vi "reorder roi.vi"(9 "Cluster Cursori":T1, 10 "Peak":i32, 11 "List ROI In in":dbl[][](array[numeric])) -> (2 "invert?":bool, 3 "List ROI In out":dbl[][](array[numeric]))   [LabVIEW 2023]
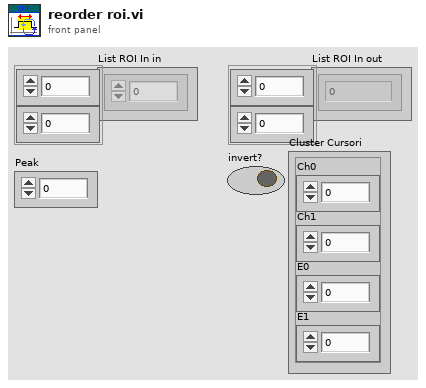
[diagram p1: front panel]
types:
  T1 = cluster{"Ch0":dbl, "Ch1":dbl, "E0":dbl, "E1":dbl}
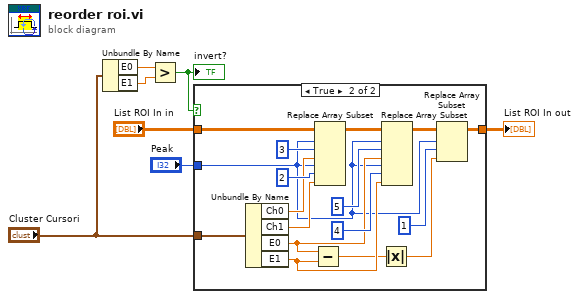
[diagram p0: block diagram]
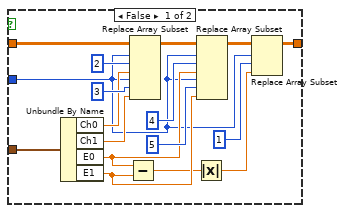
[diagram p2: hidden frame]
diagram:
  n1 = Unbundle By Name("Cluster Cursori") -> ("E0"=w2:dbl, "E1"=w1:dbl)
  n2 = Greater?(x=w2, y=w1) -> (0:w4:bool)
  "invert?" <- w4
  n3 = case shown="True" w4 {
    tunnel: "List ROI In in" -> [w24 w41]
    tunnel: [w8 w25] -> w6
    tunnel: "Peak" -> [w10 w27]
    tunnel: "Cluster Cursori" -> [w20 w37]
    frame False {
      n4 = Unbundle By Name(w20) -> ("Ch0"=w19:dbl, "Ch1"=w18:dbl, "E0"=w15:dbl, "E1"=w14:dbl)
      n5 = Subtract(x=w15, y=w14) -> (x-y=w13:dbl)
      n6 = Replace Array Subset(array=w24, new element #1=w19, index (row) #1=w10, index (col) #1=2, new element #2=w18, index (row) #2=w10, index (col) #2=3) -> (w23:dbl[][])
      n7 = Absolute Value(x=w13) -> (abs(x)=w11:dbl)
      n8 = Replace Array Subset(array=w23, new element #1=w15, index (row) #1=w10, index (col) #1=4, new element #2=w14, index (row) #2=w10, index (col) #2=5) -> (w12:dbl[][])
      n9 = Replace Array Subset(array=w12, new element=w11, index (row)=w10, index (col)=1 ("disabled index (col)")) -> (w8:dbl[][])
    }
    frame True {
      n10 = Unbundle By Name(w37) -> ("Ch0"=w36:dbl, "Ch1"=w35:dbl, "E0"=w32:dbl, "E1"=w31:dbl)
      n11 = Subtract(x=w32, y=w31) -> (x-y=w30:dbl)
      n12 = Replace Array Subset(array=w41, new element #1=w36, index (row) #1=w27, index (col) #1=3, new element #2=w35, index (row) #2=w27, index (col) #2=2) -> (w40:dbl[][])
      n13 = Absolute Value(x=w30) -> (abs(x)=w28:dbl)
      n14 = Replace Array Subset(array=w40, new element #1=w32, index (row) #1=w27, index (col) #1=5, new element #2=w31, index (row) #2=w27, index (col) #2=4) -> (w29:dbl[][])
      n15 = Replace Array Subset(array=w29, new element=w28, index (row)=w27, index (col)=1 ("disabled index (col)")) -> (w25:dbl[][])
    }
  }
  "List ROI In out" <- w6
